vi "Priority Dequeue.vi"(8 "error in (no error)":errorcluster, 9 "timeout in ms (-1)":i32=-1, 11 "Priority Queue in":refnum<class "Message Priority Queue.lvclass">) -> (0 "error out":errorcluster, 1 "timed out?":bool, 2 "element":refnum<class "Message.lvclass">, 3 "Priority Queue out":refnum<class "Message Priority Queue.lvclass">, 4 "priority":i32)   [LabVIEW 2017, in "Actor Framework.lvlib" / "Message Priority Queue.lvclass"]
uses:
  <vilib>/ActorFramework/Message Priority Queue/Message Priority Queue.lvclass
  <vilib>/ActorFramework/Message/Message.lvclass
  <vilib>/ActorFramework/Message Priority Queue/Message Priority Queue.lvclass/Message Priority Queue.ctl
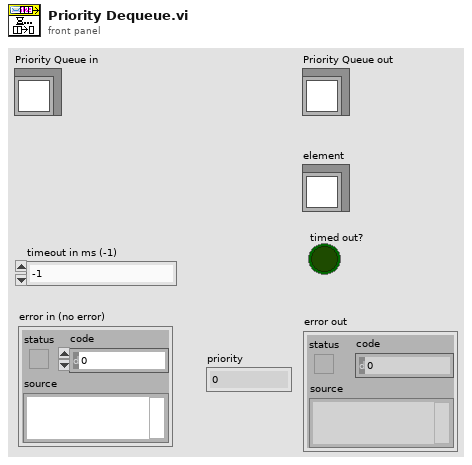
[diagram p1: front panel]
types:
  T1 = typedef "Actor Framework.lvlib/Message Priority Queue.lvclass/DVR Contents.ctl" = cluster{"# Waiting":u32, "Buffers":refnum<queue>[], "Wait Msg":refnum<queue>, "Wait Prior":refnum<queue>}
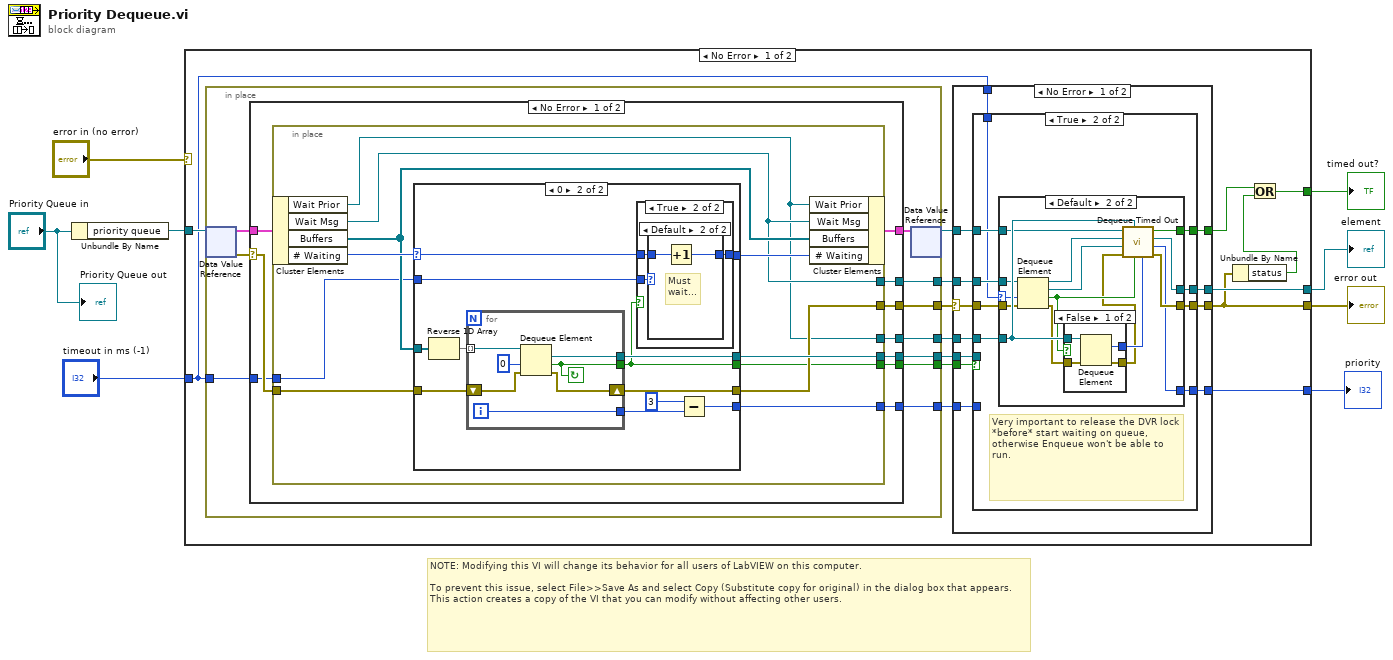
[diagram p0: block diagram]
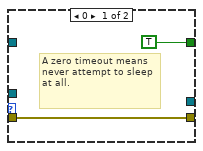
[diagram p3: hidden frame]
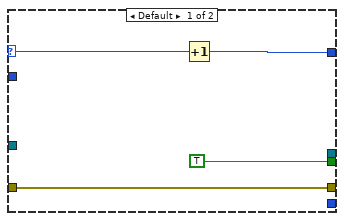
[diagram p6: hidden frame]
diagram:
  # "NOTE: Modifying this VI will change its behavior for all users of LabVIEW on this computer.\n\nTo prevent this issue, select File>>Save As and select Copy (Substitute copy for original) in the dialog box that appears. This action creates a copy of the VI that you can modify without affecting other users."
  n1 = Unbundle By Name("Priority Queue in") -> ("priority queue"=w7:refnum<data-value>)
  n2 = case shown="No Error" "error in (no error)" {
    selector: "error in (no error)" -> [_ w136]
    tunnel: [w16 w136] -> w4
    tunnel: w7 -> [w23 _]
    tunnel: [w22 _] -> w5
    tunnel: [w17 _] -> w3
    tunnel: "timeout in ms (-1)" -> [w12 _]
    tunnel: [w10 _] -> w1
    frame No Error {
      n3 = in-place {
        in-place-border: [w81] -> w13
        in-place-border: [w78] -> w21
        in-place-border: [w77] -> w20
        in-place-border: [w76] -> w19
        in-place-border: w12 -> [w75]
        in-place-border: [w74] -> w11
        in-place-border: [w73] -> w9
        n4 = in-place-dvr #1(w23) -> (w79:T1, w82:errorcluster)
        n5 = case shown="No Error" w82 {
          selector: w82 -> [w89 w135]
          tunnel: [w88 w135] -> w81
          tunnel: [w91 w134] -> w80
          tunnel: w79 -> [w92 w134]
          tunnel: [w90 _] -> w78
          tunnel: [w87 _] -> w77
          tunnel: [w86 _] -> w76
          tunnel: w75 -> [w85 _]
          tunnel: [w84 _] -> w74
          tunnel: [w83 _] -> w73
          frame No Error {
            n6 = in-place {
              in-place-border: [w103] -> w90
              in-place-border: w89 -> [w100]
              in-place-border: [w99] -> w88
              in-place-border: [w98] -> w87
              in-place-border: [w95] -> w86
              in-place-border: w85 -> [w96]
              in-place-border: [w94] -> w84
              in-place-border: [w93] -> w83
              n7 = in-place-cluster #2(w92) -> ("Wait Prior"=w94:refnum<queue>, "Wait Msg"=w95:refnum<queue>, "Buffers"=w97:refnum<queue>[], "# Waiting"=w102:u32)
              n8 = case shown="0" w102 {
                selector: w102 -> [w107 w118]
                tunnel: w97 -> [_ w119]
                tunnel: [_ w114] -> w103
                tunnel: [w106 w117] -> w101
                tunnel: w100 -> [w105 w116]
                tunnel: [w105 w115] -> w99
                tunnel: [TRUE w111] -> w98
                tunnel: w96 -> [_ w112]
                tunnel: [_ w108] -> w93
                frame Default {
                  n9 = Increment(x=w107) -> (x+1=w106:u32)
                }
                frame 0 {
                  n10 = Reverse 1D Array(array=w119) -> (reversed array=w113:refnum<queue>[])
                  n11 = for {
                    tunnel: w113 -> [w128] mode=indexing
                    tunnel: [w132] -> w111
                    shift-right: [w130] -> w115
                    shift-left: w116 -> [w131]
                    tunnel: [w129] -> w114
                    tunnel: [w127] -> w109
                    i -> [w127]
                    stop <- w132 continue-if-true
                    n12 = Dequeue Element(queue=w128, timeout in ms (-1)=0, error in (no error)=w131) -> (element=w129:refnum<class "Message.lvclass">, timed out?=w132:bool, error out=w130:errorcluster)  [unwired: 1 out]
                  }
                  n13 = case shown="True" w111 {
                    tunnel: w118 -> [w120 w123]
                    tunnel: [w120 w122] -> w117
                    tunnel: w112 -> [_ w121]
                    frame False {
                      # "Got data!\nNo need\nto wait!"
                    }
                    frame True {
                      n14 = case shown="Default" w121 {
                        tunnel: w123 -> [w124 w126]
                        tunnel: [w124 w125] -> w122
                        frame 0 {
                          # "Zero timeout does not wait."
                        }
                        frame Default {
                          # "Must \nwait..."
                          n15 = Increment(x=w126) -> (x+1=w125:u32)
                        }
                      }
                    }
                  }
                  n16 = Subtract(x=3, y=w109) -> (x-y=w108:i32)
                }
              }
              n17 = in-place-cluster #2("Wait Prior"=w94, "Wait Msg"=w95, "Buffers"=w97, "# Waiting"=w101) -> (w91:T1)
            }
          }
          frame Error {
          }
        }
        n18 = in-place-dvr #1(w80) -> (w14:refnum<data-value>)  [unwired: 1 out]
      }
      n19 = case shown="No Error" w13 {
        selector: w13 -> [w28 w72]
        tunnel: [w35 w71] -> w22
        tunnel: w21 -> [w34 w71]
        tunnel: w20 -> [w33 _]
        tunnel: w19 -> [w32 _]
        tunnel: [w31 _] -> w18
        tunnel: [w30 w72] -> w16
        tunnel: w14 -> [w29 _]
        tunnel: w12 -> [w27 _]
        tunnel: w11 -> [w26 _]
        tunnel: [w25 w70] -> w10
        tunnel: w9 -> [w24 w70]
        frame No Error {
          n20 = case shown="True" w33 {
            tunnel: [w38 w43] -> w35
            tunnel: w34 -> [w38 _]
            tunnel: w28 -> [w37 w47]
            tunnel: [w37 w42] -> w30
            tunnel: w32 -> [_ w46]
            tunnel: [_ w45] -> w31
            tunnel: w29 -> [_ w44]
            tunnel: w27 -> [_ w41]
            tunnel: w26 -> [_ w40]
            tunnel: [w36 w39] -> w25
            tunnel: w24 -> [w36 _]
            frame False {
            }
            frame True {
              # "Very important to release the DVR lock *before* start waiting on queue, otherwise Enqueue won't be able to run."
              n21 = case shown="Default" w41 {
                selector: w41 -> [_ w55]
                tunnel: w47 -> [w48 w56]
                tunnel: w46 -> [_ w63]
                tunnel: [TRUE ("really timed out?") w62] -> w45
                tunnel: w44 -> [_ w59]
                tunnel: [_ w58] -> w43
                tunnel: [w48 w57] -> w42
                tunnel: w40 -> [_ w64]
                tunnel: [_ w50] -> w39
                frame 0 {
                  # "A zero timeout means never attempt to sleep at all."
                }
                frame Default {
                  n22 = Dequeue Element(queue=w63, timeout in ms (-1)=w55, error in (no error)=w56) -> (queue out=w61:refnum<queue>, element=w60:refnum<class "Message.lvclass">, timed out?=w53:bool, error out=w52:errorcluster)
                  n23 = case shown="False" w53 {
                    tunnel: w64 -> [w68 _]
                    tunnel: [w67 _] -> w54
                    tunnel: w52 -> [w66 w69]
                    tunnel: [w65 w69] -> w51
                    frame False {
                      n24 = Dequeue Element(queue=w68, error in (no error)=w66) -> (element=w67:i32, error out=w65:errorcluster)  [unwired: 1 in, 2 out]
                    }
                    frame True {
                    }
                  }
                  n25 = call <vilib>:"Dequeue Timed Out.vi"("priority in"=w54, "timed out?"=w53, "Wait Prior"=w64, "error in (no error)"=w51, "element in"=w60, "wait queue"=w61, "priority queue"=w59) -> ("error out"=w57:errorcluster, "priority out"=w50:i32, "element out"=w58:refnum<class "Message.lvclass">, "really timed out?"=w62:bool)  [unwired: 1 in]
                }
              }
            }
          }
        }
        frame Error {
        }
      }
      n26 = Unbundle By Name(w16) -> ("status"=w15:bool)
      n27 = Or(x=w18, y=w15) -> (x .or. y?=w17:bool)
    }
    frame Error {
    }
  }
  "element" <- w5
  "error out" <- w4
  "timed out?" <- w3
  "priority" <- w1
  "Priority Queue out" <- "Priority Queue in"
